vi "Config Analog Output.vi"(0 "VISA resource name":refnum<visa-resource-name>, 1 "Mode (0:Off)":u16(ring) items=["Off", "Input", "Manual"], 2 "Source (0:Kelvin)":u16(ring) items=["Kelvin", "Celsius", "Sensor Units", "Linear Equation"], 3 "Bipolar (F: Positive Output)":bool, 5 "Analog Output (1)":dbl=1.0 min=1.0 max=2.0 step=1.0, 7 "Input (1)":dbl=1.0 min=1.0 max=8.0 step=1.0, 9 "High Value (0.0000)":dbl min=-9999.9 max=9999.9 step=0.0001 format="%.4f", 11 "error in (no error)":errorcluster, 12 "Low Value (0.0000)":dbl min=-9999.9 max=9999.9 step=0.0001 format="%.4f", 13 "Manual Value (0.0000)":dbl min=-100.0 max=100.0 step=0.0001 format="%.4f") -> (4 "VISA resource name out":refnum<visa-resource-name>, 15 "error out":errorcluster)   [LabVIEW 2017, in "Lake Shore Cryotronics 218.lvlib"]
doc: "This VI configures analog output paramters. Analog outputs may be configured manually or set to indicate the value of an input. Only the Model 218S includes the Analog Output feature."
uses:
  Lake Shore Cryotronics 218.lvlib
panel:
  # "Bipolar Output\nPositive Output"
  # "%"
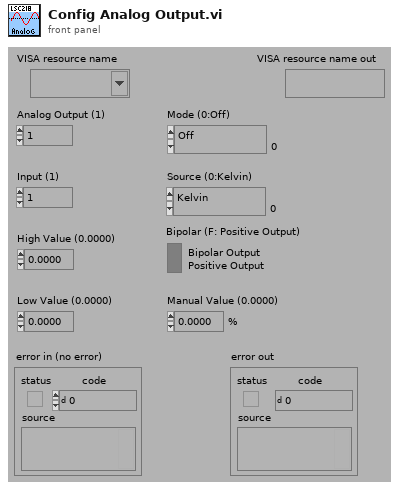
[diagram p1: front panel]
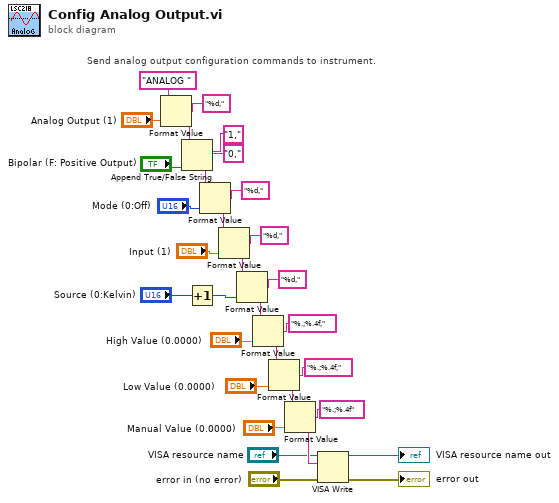
[diagram p0: block diagram]
diagram:
  # "Send analog output configuration commands to instrument."
  n1 = Format Value(string ("")="ANALOG ", format string="%d,", value (0)="Analog Output (1)") -> (output string=w19:string)
  n2 = Append True/False String(1:"Bipolar (F: Positive Output)", 2:"0,", 3:"1,", 4:w19) -> (0:w18:string)
  n3 = Increment(x="Source (0:Kelvin)") -> (x+1=w5:u16)
  n4 = Format Value(string ("")=w18, format string="%d,", value (0)="Mode (0:Off)") -> (output string=w27:string)
  n5 = Format Value(string ("")=w27, format string="%d,", value (0)="Input (1)") -> (output string=w23:string)
  n6 = Format Value(string ("")=w23, format string="%d,", value (0)=w5) -> (output string=w12:string)
  n7 = Format Value(string ("")=w12, format string="%.;%.4f,", value (0)="High Value (0.0000)") -> (output string=w11:string)
  n8 = Format Value(string ("")=w11, format string="%.;%.4f,", value (0)="Low Value (0.0000)") -> (output string=w10:string)
  n9 = Format Value(string ("")=w10, format string="%.;%.4f", value (0)="Manual Value (0.0000)") -> (output string=w9:string)
  n10 = VISA Write(VISA resource name="VISA resource name", write buffer=w9, error in (no error)="error in (no error)") -> (VISA resource name out=→"VISA resource name out":refnum<visa-resource-name>, error out=→"error out":errorcluster)  [unwired: 1 out]
